vi "WRITE - File.vi"(0 "reference in":refnum<class "TEXT.lvclass">, 5 "error in (no error)":errorcluster, 6 "Inlude Time Vector":bool, 7 "CSV Path - WRITE":path) -> (14 "reference out":refnum<class "TEXT.lvclass">, 19 "error out":errorcluster)   [LabVIEW 2020, in "TEXT.lvclass"]
uses:
  TEXT.lvclass
  API/GSwFormDSP_class/functions/Attribute List.ctl
  API/GSwFormDSP_class/GSwFormDSP.lvclass
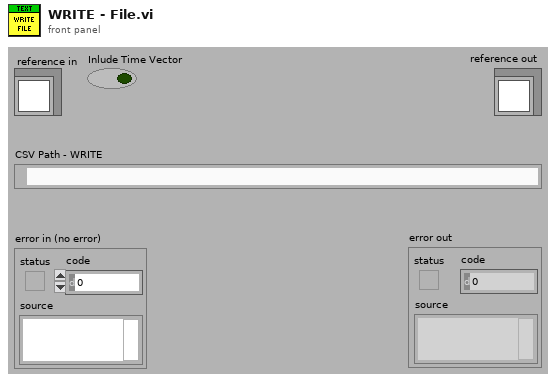
[diagram p1: front panel]
types:
  T1 = typedef "GSwFormDSP.lvclass/Attribute List.ctl" = string
  T2 = typedef "TEXT.lvclass/ObjectAttributes.ctl" = cluster{"Time Data":refnum<class "GSwFormDSP.lvclass">, "New Time Data Obj?":bool}
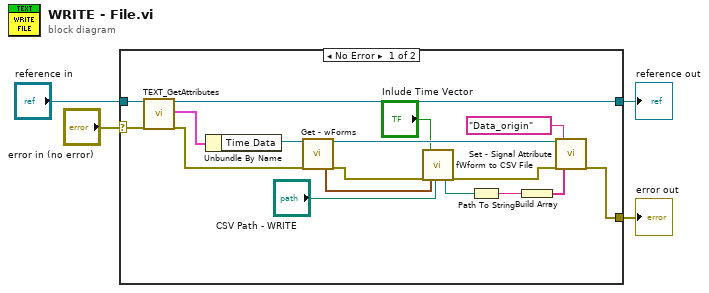
[diagram p0: block diagram]
diagram:
  n1 = case shown="No Error" "error in (no error)" {
    selector: "error in (no error)" -> [w21 w23]
    tunnel: [w14 w23] -> w3
    tunnel: [w20 w22] -> w1
    tunnel: "reference in" -> [w18 w22]
    frame No Error {
      n2 = call "TEXT_GetAttributes.vi"("reference in"=w18, "error in (no error)"=w21) -> ("reference out"=w20:refnum<class "TEXT.lvclass">, "attributes"=w19:T2, "error out"=w16:errorcluster)  [unwired: 14 in, 1 out]
      n3 = Unbundle By Name(w19) -> ("Time Data"=w17:refnum<class "GSwFormDSP.lvclass">)
      n4 = call-dynamic "Get - wForms.vi"("reference in"=w17, "error in (no error)"=w16) -> ("wForms"=w11:waveform(dbl)[], "reference out"=w15:refnum<class "GSwFormDSP.lvclass">, "error out"=w13:errorcluster)  [unwired: 14 in, 1 out]
      n5 = call "fWform to CSV File.vi"("error in (no error)"=w13, "Inlude Time Vector"="Inlude Time Vector", "wForms"=w11, "CSV Path IN"="CSV Path - WRITE") -> ("CSV Path OUT"=w9:path, "error out"=w12:errorcluster)  [unwired: 14 in]
      n6 = Path To String(path=w9) -> (string=w8:string)
      n7 = Build Array(w8) -> (w7:string[])
      n8 = call-dynamic "Set - Signal Attribute.vi"("reference in"=w15, "error in (no error)"=w12, "wForm Attributes"=T1 "Data_origin", "Attribute"=w7) -> ("error out"=w14:errorcluster)  [unwired: 14 in, 1 out]
    }
    frame Error {
    }
  }
  "error out" <- w3
  "reference out" <- w1
